vi "Fft.vi"   [LabVIEW 2015]
uses:
  <vilib>/Platform/TimedLoop/XDataNode/timing_clust.ctl
  <vilib>/Platform/TimedLoop/XDataNode/nitl_modes.ctl
  <vilib>/Platform/TimedLoop/XDataNode/wakeup.ctl
  <vilib>/rvi/Analysis/measure/FFT/simModelSupport/niFPGA FFT Sim Properties.ctl
  <vilib>/rvi/Analysis/measure/FFT/simModelSupport/niFPGA FFT Sim Types.ctl
  <vilib>/rvi/Analysis/measure/FFT/simModelSupport/niFpgaFFTSimArithmeticProperties.ctl
  <vilib>/rvi/Analysis/measure/FFT/simModelSupport/niFpgaFFTSimDfxp.ctl
  <vilib>/fxp/LVFixedPointQuantizationPolicyTypeDef.ctl
  <vilib>/rvi/Emulation/niFpgaSctlEmulationGetInTimedLoop.vi
  <vilib>/rvi/Emulation/niFpgaEmulationReportErrorSimple.vi
  <vilib>/rvi/Emulation/niFpgaGetClockAttributes.vi
  <vilib>/rvi/Emulation/niFpgaCriticalErrorInLSC.vi
  <vilib>/rvi/interface/RandomDataEmulation/niFpgaRandomDataHandleErrors.vi
  <vilib>/rvi/Emulation/niFpgaEmulationIsFPGAContextNoSignature.vi
  <vilib>/rvi/errors/niFpgaSetErrorForExecOnDevCompSimple.vi
  <vilib>/rvi/eio/common/nirviEmuReportErrorAndStop.vi
  <vilib>/rvi/DataTransferAndStorage/Container/Common/niFpgaContainerGetUniqueNameForEmu.vi
  <vilib>/rvi/FIFO/Fifo_Resource/nirvififoEmulationSetSize.vi
  <vilib>/rvi/FIFO/Fifo_Resource/nirviFifoEmulationQueueMgr.vi
  <instcachedir>/0/nirviFifoEmulationQueueMgr_E5CAEC123FF24DC58D834DCA3CDAA9B5.lvgen/nirviFifoEmulationQueueMgr_E5CAEC123FF24DC58D834DCA3CDAA9B5_001.vi
  <vilib>/rvi/FIFO/Fifo_Resource/nirvififoEmulationDetermineInputValidOut.vi
  <vilib>/rvi/FIFO/Fifo_Resource/nirvififoEmulationCreateLock.vi
  <vilib>/rvi/Emulation/niFpgaProcessEmulError.vi
  <vilib>/rvi/FIFO/Fifo_Resource/nirvififoEmulationObtainLock.vi
  <vilib>/rvi/FIFO/Fifo_Resource/nirvififoEmulationReleaseLock.vi
  <vilib>/rvi/occurrence/nirviWaitOnOccurrenceBase.vi
  <vilib>/rvi/errors/nirviReportUnexpectedCaseInternalError.vi
  <vilib>/rvi/errors/nirviReportUnexpectedCaseInternalError (U32).vi
  <vilib>/Utility/error.llb/Clear Errors.vi
  <vilib>/rvi/Analysis/measure/FFT/simModelSupport/niFpgaFFTSimModelCore.vi
  <vilib>/Platform/TimedLoop/XDataNode/XDataNode.xnode
  <vilib>/rvi/DataTransferAndStorage/Container/XNode/niFpgaContainer.xnode
  <vilib>/rvi/interface/RandomDataEmulation/nirviRandomDataFpgaReadWriteTemplate.vi
  <vilib>/rvi/FIFO/Fifo_Resource/nirvififoEmulationWrite.vi
  <vilib>/rvi/FIFO/Fifo_Resource/nirvififoEmulationRead.vi
  <vilib>/rvi/Analysis/measure/FFT/XNode/niFpgaFFT.xnode
  <vilib>/Platform/TimedLoop/XDataNode/XDNodeRunTimeDep.lvlib
types:
  T1 = typedef "XDNodeRunTimeDep.lvlib/timing_clust.ctl" = cluster{"Expected End [f-1]":u64, "Actual End [f-1]":u64, "Finished Late? [f-1]":bool, "Expected End [i-1]":u64, "Actual End [i-1]":u64, "Finished Late? [i-1]":bool, "Expected Start [i]":u64, "Actual Start [i]":u64, "Expected Start [f]":u64, "Actual Start [f]":u64, "Source Name":string, "Structure Name":string, "Period":i64, "Deadline":i64, "Offset":i64, "Start":i64, "Priority":i32, "Timeout":i32, "Mode":T2, "Wakeup Reason":T3, "Error":errorcluster, "Source Type":string, "Secondary Source Type":string, "Global End Time":u64, "Global Start Time":u64, "Frame Duration":u64, "Iteration Duration":u64, "Assigned CPU":i32, "I/O Scan Engine Mode":u32}
  T2 = typedef "XDNodeRunTimeDep.lvlib/nitl_modes.ctl" = enum32{"No Change", "Process missed periods, maintain original phase", "Discard missed periods, maintain original phase", "Process missed periods, ignore original phase", "Discard missed periods, ignore original phase"}
  T3 = typedef "XDNodeRunTimeDep.lvlib/wakeup.ctl" = enum32{"Normal", "Aborted", "Asynchronous wakeup", "Timing source error", "Timed loop error", "Timeout"}
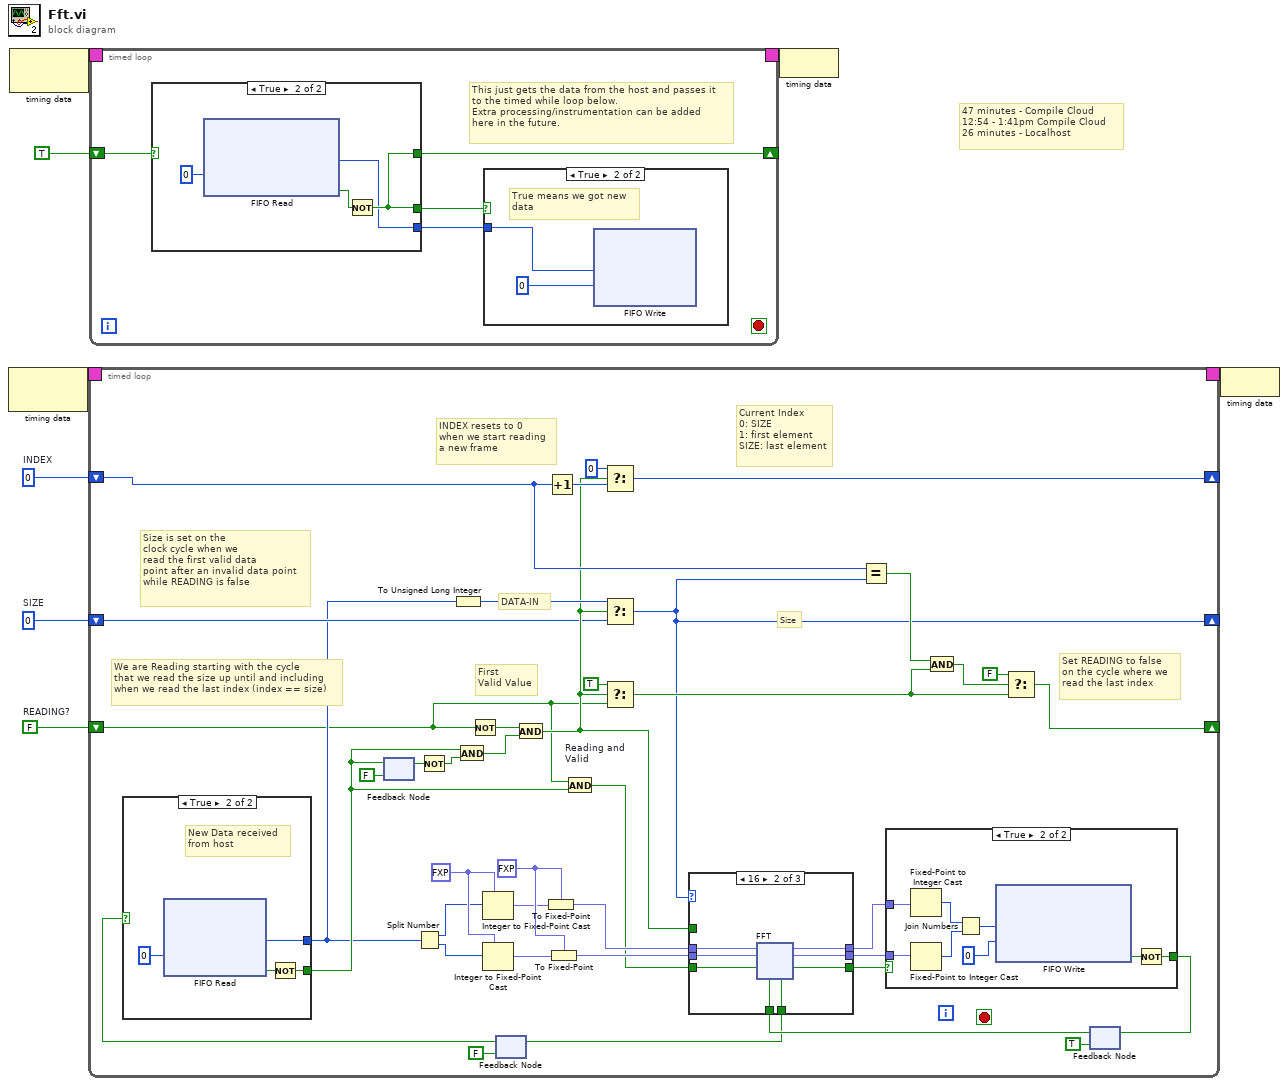
[diagram p0: block diagram]
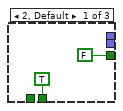
[diagram p2: hidden frame]
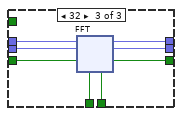
[diagram p3: hidden frame]
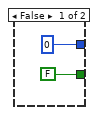
[diagram p4: hidden frame]
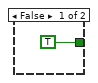
[diagram p5: hidden frame]
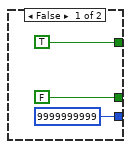
[diagram p7: hidden frame]
diagram:
  w1 = u32 0  # INDEX
  w2 = FALSE  # READING?
  w3 = u32 0  # SIZE
  # "47 minutes - Compile Cloud\n12:54 - 1:41pm Compile Cloud\n26 minutes - Localhost"
  n1 = node-c288() -> (w5:T1)  [unwired: 1 in]
  n2 = node-c288() -> (w8:T1)  [unwired: 1 in]
  n3 = timed-loop {
    timing: w5 -> [_]
    timing-out: [_] -> w4
    shift-right: [w10] -> _
    shift-left: w3 -> [w17]
    shift-right: [w12] -> _
    shift-left: w2 -> [w9]
    shift-right: [w26] -> _
    shift-left: w1 -> [w24]
    stop <- _ stop-if-true
    w42 = fxp<+/-,24,7> 0.0 ("real data in")
    w44 = fxp<+/-,32,7> 0.0 ("real data in")
    # "Set READING to false\non the cycle where we\nread the last index"
    # "Current Index\n0: SIZE\n1: first element\nSIZE: last element"
    # "INDEX resets to 0\nwhen we start reading\na new frame"
    # "We are Reading starting with the cycle\nthat we read the size up until and including\nwhen we read the last index (index == size)"
    # "Size is set on the \nclock cycle when we\nread the first valid data\npoint after an invalid data point\nwhile READING is false"
    # "First\nValid Value"
    # "DATA-IN"
    # "Size"
    n4 = feedback #1(FALSE ("Timed Out?")) -> (w36:bool)
    n5 = Not(x=w36) -> (.not. x?=w35:bool)
    n6 = Not(x=w9) -> (.not. x?=w33:bool)
    n7 = feedback #2(FALSE ("ready for data")) -> (w22:bool)
    n8 = case shown="True" w22 {
      tunnel: [FALSE ("Timed Out?") w124] -> w20
      tunnel: [u64 0 ("Element") w121] -> w13
      frame False {
      }
      frame True {
        # "New Data received \nfrom host"
        n9 = xnode ("FIFO Read")("Timeout"=0) -> ("Element"=w121:u64, "Timed Out?"=w122:bool)  [unwired: 1 in, 1 out]
        n10 = Not(x=w122) -> (.not. x?=w124:bool)
      }
    }
    n11 = feedback-in #1(w20) -> ()
    n12 = Split Number(x=w13) -> (hi(x)=w43:u32, lo(x)=w47:u32)
    n13 = To Unsigned Long Integer(number=w13) -> (unsigned 32bit integer=w34:u32)
    n14 = And(x=w20, y=w35) -> (x .and. y?=w21:bool)
    n15 = Integer to Fixed-Point Cast(fixed-point type=w44, integer=w43) -> (fixed-point=w40:fxp<+/-,32,7>)
    n16 = Integer to Fixed-Point Cast(fixed-point type=w44, integer=w47) -> (fixed-point=w41:fxp<+/-,32,7>)
    n17 = And(x=w33, y=w21) -> (x .and. y?=w19:bool)
    n18 = To Fixed-Point(fixed-point type=w42, number=w40) -> (fixed-point=w27:fxp<+/-,24,7>)
    n19 = Increment(x=w24) -> (x+1=w30:u32)
    n20 = To Fixed-Point(fixed-point type=w42, number=w41) -> (fixed-point=w28:fxp<+/-,24,7>)
    n21 = And "Reading and\nValid"(x=w9, y=w20) -> (x .and. y?=w11:bool)
    n22 = Select(t=u32 0, s=w19, f=w30) -> (s? t:f=w26:u32)
    n23 = Select(t=w34, s=w19, f=w17) -> (s? t:f=w10:u32)
    n24 = Select(t=TRUE, s=w19, f=w9) -> (s? t:f=w18:bool)
    n25 = Equal?(x=w24, y=w10) -> (x = y?=w25:bool)
    n26 = And(x=w25, y=w18) -> (x .and. y?=w23:bool)
    n27 = Select(t=FALSE, s=w23, f=w18) -> (s? t:f=w12:bool)
    n28 = feedback #3(TRUE ("Timed Out?")) -> (w16:bool)
    n29 = case shown="16" w10 {
      tunnel: [TRUE ("ready for input") w54 w85] -> w14
      tunnel: w16 -> [_ w58 w92]
      tunnel: w28 -> [_ w57 w91]
      tunnel: w27 -> [_ w51 w90]
      tunnel: [FALSE ("output valid") w52 w89] -> w39
      tunnel: [_ w56 w88] -> w15
      tunnel: [_ w55 w87] -> w38
      tunnel: w11 -> [_ w53 w86]
      tunnel: w19 -> [_ _ _]
      frame 2, Default {
      }
      frame 16 {
        n30 = xnode "FFT"("real data in"=w51, "imaginary data in"=w57, "input valid"=w53, "ready for output"=w58) -> ("ready for input"=w54:bool, "real data out"=w56:fxp<+/-,32,12>, "imaginary data out"=w55:fxp<+/-,32,12>, "output valid"=w52:bool)  [unwired: 1 in, 1 out]
      }
      frame 32 {
        n31 = xnode "FFT"("real data in"=w90, "imaginary data in"=w91, "input valid"=w86, "ready for output"=w92) -> ("ready for input"=w85:bool, "real data out"=w88:fxp<+/-,32,13>, "imaginary data out"=w87:fxp<+/-,32,13>, "output valid"=w89:bool)  [unwired: 1 in, 1 out]
      }
    }
    n32 = feedback-in #2(w14) -> ()
    n33 = case shown="True" w39 {
      tunnel: w15 -> [_ w126]
      tunnel: w38 -> [_ w131]
      tunnel: [TRUE ("Timed Out?") w127] -> w46
      frame False {
      }
      frame True {
        n34 = Fixed-Point to Integer Cast(1:w126) -> (0:w133:i64)
        n35 = Fixed-Point to Integer Cast(1:w131) -> (0:w132:i64)
        n36 = Join Numbers(hi=w133, lo=w132) -> ((hi.lo)=w130:u64)
        n37 = xnode ("FIFO Write")("Element"=w130, "Timeout"=0) -> ("Timed Out?"=w128:bool)  [unwired: 1 in, 1 out]
        n38 = Not(x=w128) -> (.not. x?=w127:bool)
      }
    }
    n39 = feedback-in #3(w46) -> ()
  }
  n40 = timed-loop {
    timing: w8 -> [_]
    timing-out: [_] -> w7
    shift-right: [w137] -> _
    shift-left: TRUE -> [w139]
    stop <- _ stop-if-true
    # "This just gets the data from the host and passes it\nto the timed while loop below.\nExtra processing/instrumentation can be added\nhere in the future."
    n41 = case shown="True" w139 {
      tunnel: [TRUE w148] -> w137
      tunnel: [u64 9999999999 ("Element") w145] -> w138
      tunnel: [FALSE w148] -> w136
      frame False {
      }
      frame True {
        n42 = xnode ("FIFO Read")("Timeout"=0) -> ("Element"=w145:u64, "Timed Out?"=w146:bool)  [unwired: 1 in, 1 out]
        n43 = Not(x=w146) -> (.not. x?=w148:bool)
      }
    }
    n44 = case shown="True" w136 {
      tunnel: w138 -> [_ w140]
      frame False {
      }
      frame True {
        # "True means we got new\ndata"
        n45 = xnode ("FIFO Write")("Element"=w140, "Timeout"=0) -> ()  [unwired: 1 in, 2 out]
      }
    }
  }
  n46 = node-c288(w7) -> ()
  n47 = node-c288(w4) -> ()
